vi "Tacho_and_Force_Calibration.vi"(9 "Force Ref In":T1, 10 "Tacho Ref In":T1, 11 "Calibration_Length":i32) -> (2 "Force_calib_value":dbl, 3 "Velocity_calib_value":dbl)   [LabVIEW 2019]
uses:
  <vilib>/myRIO/Instrument Drivers/Onboard IO/AI/typedefs/AI Reference.ctl
  <vilib>/myRIO/Common/Instrument Driver Framework/Utilities/typedefs/myRIO Generic Hardware Reference.ctl
  <vilib>/myRIO/Common/Instrument Driver Framework/Utilities/typedefs/Hardware Version Enum.ctl
  <vilib>/myRIO/Common/Instrument Driver Framework/Utilities/typedefs/myRIO v1.0 Reference.ctl
  <vilib>/myRIO/Common/Instrument Driver Framework/Utilities/typedefs/Generic FPGA Reference.ctl
  <vilib>/myRIO/Common/Instrument Driver Framework/myRIO v1.0/AI/typedefs/AI Channels List.ctl
  <vilib>/myRIO/Common/Instrument Driver Framework/myRIO v1.0/AI/typedefs/AI Channels Enum.ctl
  <vilib>/myRIO/Common/Instrument Driver Framework/Utilities/typedefs/Analog Scaling Constants List.ctl
  <vilib>/myRIO/Common/Instrument Driver Framework/Utilities/typedefs/Analog Scaling Constants.ctl
  <vilib>/Utility/error.llb/Error Cluster From Error Code.vi
  <vilib>/myRIO/Common/Instrument Driver Framework/myRIO v1.0/AI/vis/myRIO v1.0 Read AI.vi
  <vilib>/myRIO/Instrument Drivers/Onboard IO/AI/AI.lvlib
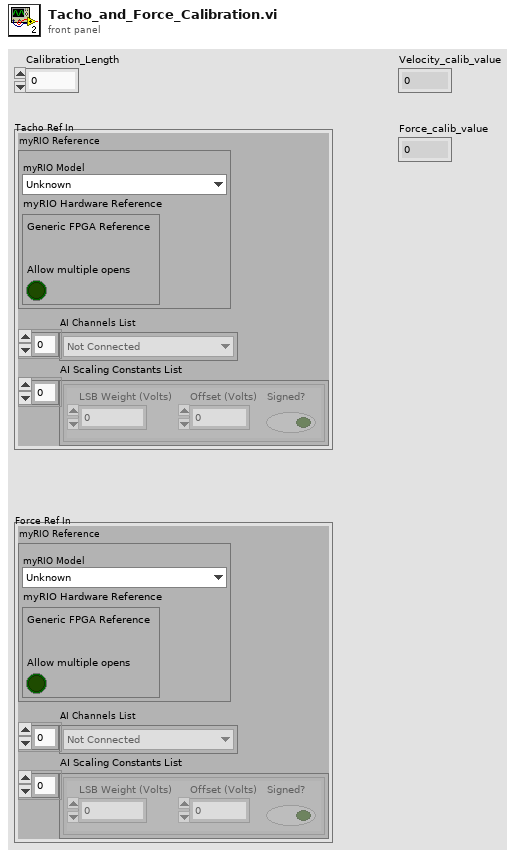
[diagram p1: front panel]
types:
  T1 = typedef "AI.lvlib/AI Reference.ctl" = cluster{"myRIO Reference":T2, "AI Channels List":T6, "AI Scaling Constants List":T8}
  T2 = typedef "myRIO Generic Hardware Reference.ctl" = cluster{"myRIO Model":T3, "myRIO Hardware Reference":T4}
  T3 = typedef "Hardware Version Enum.ctl" = enum16{"Unknown", "myRIO-1900", "myRIO-1950", "roboRIO", "NI ELVIS RIO CM", "ELVIS III"}
  T4 = typedef "myRIO v1.0 Reference.ctl" = cluster{"Generic FPGA Reference":T5, "Allow multiple opens":bool}
  T5 = typedef "Generic FPGA Reference.ctl" = refnum<k20>
  T6 = typedef "AI Channels List.ctl" = T7[]
  T7 = typedef "AI Channels Enum.ctl" = enum16{"Not Connected", "AudioIn/Left", "AudioIn/Right", "C/AI0", "C/AI1", "A/AI0", "A/AI1", "A/AI2", "A/AI3", "A/AI4", "A/AI5", "A/AI6", "A/AI7", "B/AI0", "B/AI1", "B/AI2", "B/AI3", "B/AI4", "B/AI5", "B/AI6", "B/AI7", "AI/AI0", "AI/AI1", "AI/AI2", "AI/AI3", "A/AI0 (DIFF)", "A/AI1 (DIFF)", "A/AI2 (DIFF)", "A/AI3 (DIFF)", "B/AI0 (DIFF)", "B/AI1 (DIFF)", "B/AI2 (DIFF)", "B/AI3 (DIFF)"}
  T8 = typedef "Analog Scaling Constants List.ctl" = T9[]
  T9 = typedef "Analog Scaling Constants.ctl" = cluster{"LSB Weight (Volts)":dbl, "Offset (Volts)":dbl, "Signed?":bool}
  T10 = typedef "TypeDefTachometerParam.ctl" = cluster{"Offset [V]":dbl, "Gain [deg/sV]":dbl}
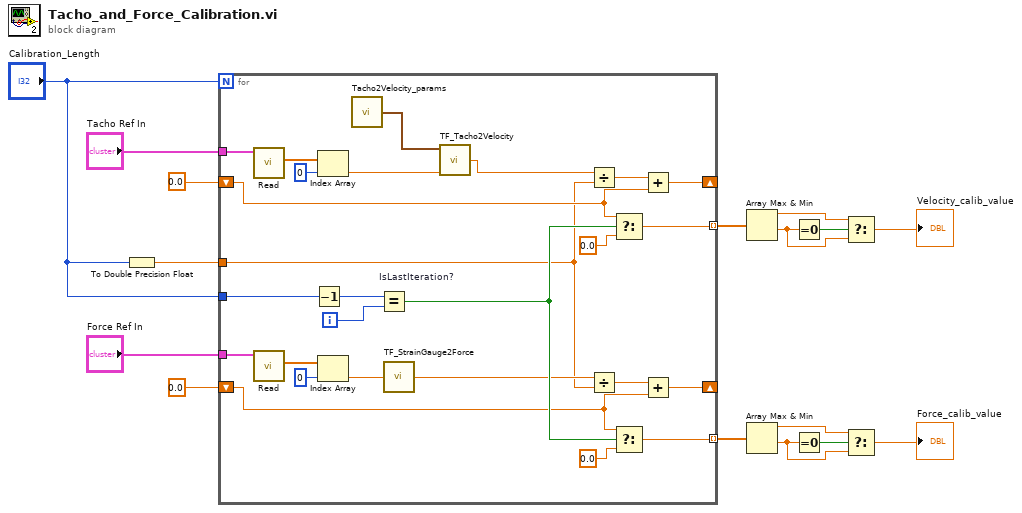
[diagram p0: block diagram]
diagram:
  n1 = To Double Precision Float(number="Calibration_Length") -> (double precision float=w1:dbl)
  n2 = for {
    N: "Calibration_Length" -> [_]
    tunnel: "Force Ref In" -> [w40]
    shift-right: [w39] -> _
    shift-left: 0.0 -> [w23]
    tunnel: [w37] -> w4 mode=indexing
    tunnel: "Tacho Ref In" -> [w34]
    shift-right: [w32] -> _
    shift-left: 0.0 -> [w22]
    tunnel: [w28] -> w15 mode=indexing
    tunnel: "Calibration_Length" -> [w21]
    tunnel: w1 -> [w20]
    i -> [w31]
    n3 = call <vilib>:"Read.vi"("AI Ref In"=w34) -> ("Values"=w36:dbl[])  [unwired: 8 in, 2 out]
    n4 = call <vilib>:"Read.vi"("AI Ref In"=w40) -> ("Values"=w41:dbl[])  [unwired: 8 in, 2 out]
    n5 = Decrement(x=w21) -> (x-1=w25:i32)
    n6 = Index Array(array=w36, index=0) -> (element=w18:dbl)
    n7 = Index Array(array=w41, index=0) -> (element=w27:dbl)
    n8 = call "Tacho2Velocity_params.vi"() -> ("Cluster"=w19:T10)  [unwired: 5 in]
    n9 = Equal? "IsLastIteration?"(x=w25, y=w31) -> (x = y?=w30:bool)
    n10 = call "TF_StrainGauge2Force.vi"("Strain Gauge Value [V]"=w27) -> ("Force [N]"=w26:dbl)  [unwired: 4 in]
    n11 = call "TF_Tacho2Velocity.vi"("Tachometer Voltage [V]"=w18, "Tachometer param"=w19) -> ("Tachometer Velocity [deg/s]"=w17:dbl)  [unwired: 2 in]
    n12 = Divide(x=w17, y=w20) -> (x/y=w33:dbl)
    n13 = Divide(x=w26, y=w20) -> (x/y=w24:dbl)
    n14 = Select(t=w22, s=w30, f=0.0) -> (s? t:f=w28:dbl)
    n15 = Select(t=w23, s=w30, f=0.0) -> (s? t:f=w37:dbl)
    n16 = Add(x=w33, y=w22) -> (x+y=w32:dbl)
    n17 = Add(x=w24, y=w23) -> (x+y=w39:dbl)
  }
  n18 = Array Max & Min(array=w15) -> (max value=w13:dbl, min value=w14:dbl)  [unwired: 2 out]
  n19 = Array Max & Min(array=w4) -> (max value=w7:dbl, min value=w8:dbl)  [unwired: 2 out]
  n20 = Equal To 0?(x=w14) -> (x = 0?=w12:bool)
  n21 = Equal To 0?(x=w8) -> (x = 0?=w6:bool)
  n22 = Select(t=w13, s=w12, f=w14) -> (s? t:f=→"Velocity_calib_value":dbl)
  n23 = Select(t=w7, s=w6, f=w8) -> (s? t:f=→"Force_calib_value":dbl)
